vi "Next Month.vi"(5 "month in":u16) -> (2 "month out":u16)   [LabVIEW 2020]
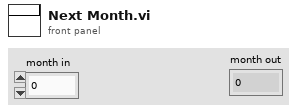
[diagram p1: front panel]
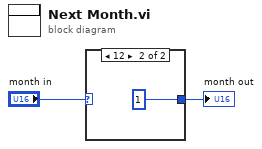
[diagram p0: block diagram]
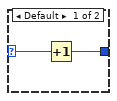
[diagram p2: hidden frame]
diagram:
  n1 = case shown="12" "month in" {
    selector: "month in" -> [w4 _]
    tunnel: [w3 u16 1] -> w1
    frame Default {
      n2 = Increment(x=w4) -> (x+1=w3:u16)
    }
    frame 12 {
    }
  }
  "month out" <- w1
